vi "filter.release.week.vi"(10 "date":timestamp, 11 "manager_daemon in":refnum<class "manager_daemon.lvclass">) -> (2 "volume sortable_names":string[](array[string]), 3 "manager_daemon out":refnum<class "manager_daemon.lvclass">)   [LabVIEW 2024, in "manager_daemon.lvclass"]
uses:
  manager_daemon.lvclass
  manager_daemon.lvclass/manager_daemon.ctl
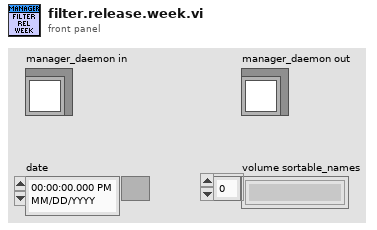
[diagram p1: front panel]
types:
  T1 = typedef "manager_daemon.lvclass/VolumeData--cluster.ctl" = cluster{"name":string, "sortable_name":string, "aliases":string[], "description":string, "site_detail_url":string, "count_of_issues":i32, "start_year":i32, "publisher_id":i32, "issue_ids":i32[], "date_last_updated":timestamp, "volume":i32, "cv_id":string, "volume type":T2, "source_path":path}
  T2 = typedef "CV_Shared_Library.lvlib/volume.type--enum.ctl" = enum16{"Ongoing", "Limited Series", "Annual", "One Shot", "Reprint/Document", "Star Comics", "Epic Comics"}
  T3 = typedef "manager_daemon.lvclass/IssueData--clustrer.ctl" = cluster{"cover_date":timestamp, "cv_id":string, "name":string, "sortable_name":string, "issue_number":string, "deck":string, "description":string, "volume id":i32, "store_date":timestamp, "date_last_updated":timestamp, "site_detail_url":string, "cover_url":string, "source_path":path, "in_collection":bool}
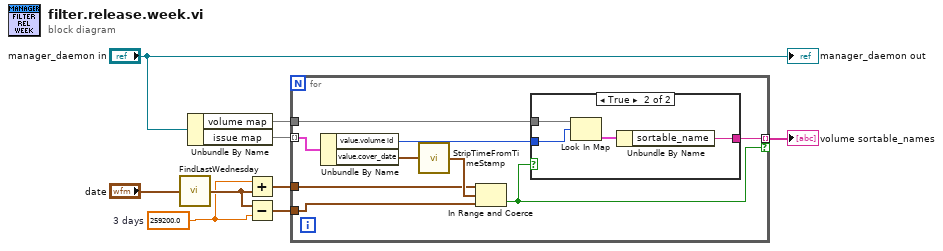
[diagram p0: block diagram]
diagram:
  w3 = 259200.0  # 3 days
  n1 = call "FindLastWednesday.vi"("current time"="date") -> ("Most Recent Wednesday"=w4:timestamp)
  n2 = Unbundle By Name("manager_daemon in") -> ("volume map"=w7:map{i32, T1}, "issue map"=w9:map{i32, T3})
  n3 = Add(x=w3, y=w4) -> (x+y=w1:timestamp)
  n4 = Subtract(x=w4, y=w3) -> (x-y=w2:timestamp)
  n5 = for {
    tunnel: w9 -> [w18] mode=indexing
    tunnel: w7 -> [w16]
    tunnel: [w14] -> w6 mode=indexing if=w13
    tunnel: w2 -> [w11]
    tunnel: w1 -> [w10]
    n6 = Unbundle By Name(w18) -> ("value.volume id"=w15:i32, "value.cover_date"=w17:timestamp)
    n7 = call "StripTimeFromTimeStamp.vi"("current time"=w17) -> ("date only"=w12:timestamp)  [unwired: 4 in]
    n8 = In Range and Coerce(upper limit=w10, x=w12, lower limit=w11) -> (In Range?=w13:bool)  [unwired: 1 out]
    n9 = case shown="True" w13 {
      tunnel: w16 -> [_ w22]
      tunnel: w15 -> [_ w21]
      tunnel: [_ w19] -> w14
      frame False {
      }
      frame True {
        n10 = Look In Map(map=w22, key=w21) -> (value=w20:T1)  [unwired: 1 in, 1 out]
        n11 = Unbundle By Name(w20) -> ("sortable_name"=w19:string)
      }
    }
  }
  "volume sortable_names" <- w6
  "manager_daemon out" <- "manager_daemon in"
